vi "XML Script - SubVI.vi"   [LabVIEW 2017]
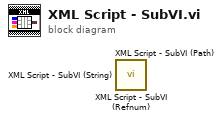
[diagram p0: block diagram]
diagram:
  n1 = call <vilib>:"XML Script - SubVI (Refnum).vi"() -> ()  [unwired: 10 in, 2 out]
  n2 = call <vilib>:"XML Script - SubVI (Path).vi"() -> ()  [unwired: 10 in, 2 out]
  n3 = call <vilib>:"XML Script - SubVI (String).vi"() -> ()  [unwired: 10 in, 2 out]
